vi "Process Image.vi"(8 "error in (no error)":errorcluster, 10 "Image Analysis IN":T1, 11 "Cluster in":T3={"Draw Xhair IN "={"Draw"=TRUE, "Target"={"x"=20.0, "y"=20.0}, "Size"={"x"=20.0, "y"=20.0}, "Angle"=1250067.0, "Color"=1250067, "Thickness"=20, "CrosshairLabel"=""}, "Autoscale"=FALSE, "Scale"={"scale factor"=0.0, "Scale"=FALSE}, "Lowpass IN"={"LowPass"=FALSE, "Size & Tolerance"={"X Size"=0, "Y Size"=0, "% Tolerance"=0}}, "Image"=refnum, "GUI_centroid overlay"={"CentroidX array"=[], "CentroidY array"=[], "CentroidX"=0.0, "CentroidY"=0.0, "# images to average"=1250067, "Overlay Size"={"xhair size"=0.0, "xhair size 2"=0.0}, "Color"=1250067, "Draw"=FALSE, "Thickness"=0}, "GUI Xhair"={"Draw"=TRUE, "Target"={"x"=20.0, "y"=20.0}, "Size"={"x"=20.0, "y"=20.0}, "Angle"=1250067.0, "Color"=1250067, "Thickness"=20, "CrosshairLabel"=""}} {"Draw Xhair IN"."Thickness" max=0; "Draw Xhair IN"."Target"."y" min=0.0 max=0.0; "Draw Xhair IN"."Target"."x" min=0.0 max=0.0; "Draw Xhair IN"."Angle" format="%#_13g"; "Draw Xhair IN"."Size"."y" min=0.0 max=0.0; "Draw Xhair IN"."Size"."x" min=0.0 max=0.0; "GUI Xhair"."Thickness" max=0; "GUI Xhair"."Target"."y" min=0.0 max=0.0; "GUI Xhair"."Target"."x" min=0.0 max=0.0; "GUI Xhair"."Angle" format="%#_13g"; "GUI Xhair"."Size"."y" min=0.0 max=0.0; "GUI Xhair"."Size"."x" min=0.0 max=0.0}) -> (0 "error out":errorcluster, 2 "Image Analysis OUT":T1, 3 "Cluster out":T3={"Draw Xhair IN "={"Draw"=TRUE, "Target"={"x"=20.0, "y"=20.0}, "Size"={"x"=20.0, "y"=20.0}, "Angle"=1250067.0, "Color"=1250067, "Thickness"=20, "CrosshairLabel"=""}, "Autoscale"=FALSE, "Scale"={"scale factor"=0.0, "Scale"=FALSE}, "Lowpass IN"={"LowPass"=FALSE, "Size & Tolerance"={"X Size"=0, "Y Size"=0, "% Tolerance"=0}}, "Image"=refnum, "GUI_centroid overlay"={"CentroidX array"=[], "CentroidY array"=[], "CentroidX"=0.0, "CentroidY"=0.0, "# images to average"=1250067, "Overlay Size"={"xhair size"=0.0, "xhair size 2"=0.0}, "Color"=1250067, "Draw"=FALSE, "Thickness"=0}, "GUI Xhair"={"Draw"=TRUE, "Target"={"x"=20.0, "y"=20.0}, "Size"={"x"=20.0, "y"=20.0}, "Angle"=1250067.0, "Color"=1250067, "Thickness"=20, "CrosshairLabel"=""}} {"Draw Xhair IN"."Thickness" max=0; "Draw Xhair IN"."Target"."y" min=0.0 max=0.0; "Draw Xhair IN"."Target"."x" min=0.0 max=0.0; "Draw Xhair IN"."Angle" format="%#_13g"; "Draw Xhair IN"."Size"."y" min=0.0 max=0.0; "Draw Xhair IN"."Size"."x" min=0.0 max=0.0; "GUI Xhair"."Thickness" max=0; "GUI Xhair"."Target"."y" min=0.0 max=0.0; "GUI Xhair"."Target"."x" min=0.0 max=0.0; "GUI Xhair"."Angle" format="%#_13g"; "GUI Xhair"."Size"."y" min=0.0 max=0.0; "GUI Xhair"."Size"."x" min=0.0 max=0.0})   [LabVIEW 2020]
uses:
  Controls/Image Processing Controls.ctl
  General GUIs/Device GUIs/GUI_Cameras/Controls/Crosshair type def.ctl
  <vilib>/vision/Image Controls.llb/IMAQ Image.ctl
  Controls/GUI_running average centroid overlay.ctl
  Controls/Image Analysis Controls.ctl
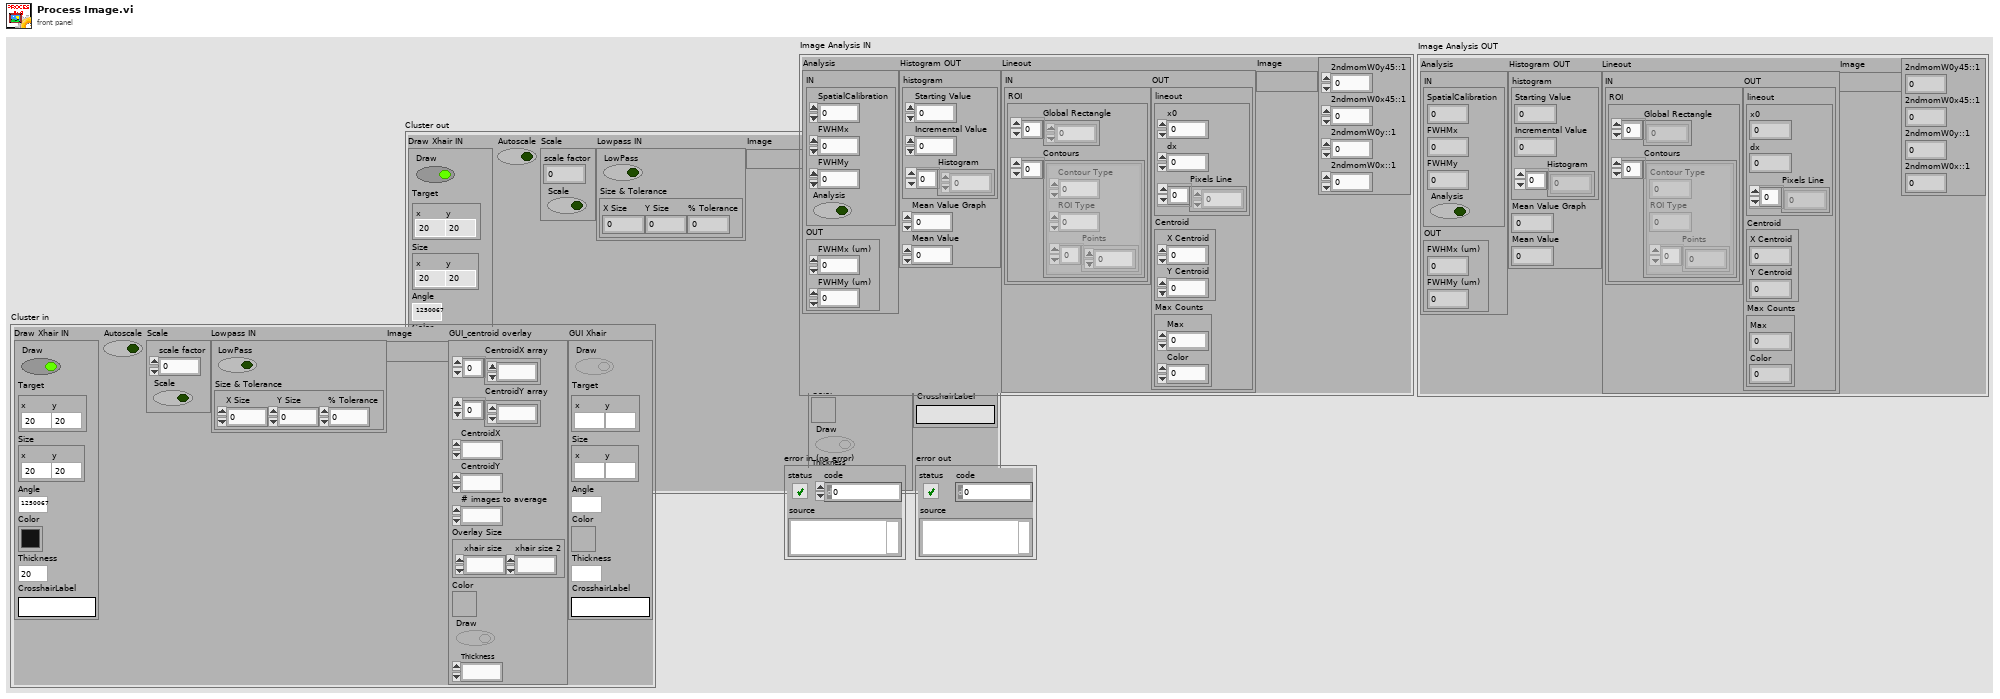
[diagram p1: front panel]
types:
  T1 = typedef "Image Analysis Controls.ctl" = cluster{"Analysis":cluster{"IN":cluster{"SpatialCalibration":dbl, "FWHMx":dbl, "FWHMy":dbl, "Analysis":bool}, "OUT":cluster{"FWHMx (um)":dbl, "FWHMy (um)":dbl}}, "Histogram OUT":cluster{"histogram":cluster{"Starting Value":sgl, "Incremental Value":sgl, "Histogram":u32[]}, "Mean Value Graph":sgl, "Mean Value":sgl}, "Lineout":cluster{"IN":cluster{"ROI":cluster{"Global Rectangle":i32[], "Contours":cluster{"Contour Type":u32, "ROI Type":u32, "Points":i32[]}[]}}, "OUT":cluster{"lineout":cluster{"x0":sgl, "dx":sgl, "Pixels Line":sgl[]}, "Centroid":cluster{"X Centroid":sgl, "Y Centroid":sgl}, "Max Counts":cluster{"Max":sgl, "Color":u32}}}, "Image":T2, "variables":cluster{"2ndmomW0y45::1":dbl, "2ndmomW0x45::1":dbl, "2ndmomW0y::1":dbl, "2ndmomW0x::1":dbl}}
  T2 = typedef "IMAQ Image.ctl" = refnum<image>
  T3 = typedef "Image Processing Controls.ctl" = cluster{"Draw Xhair IN ":T4, "Autoscale":bool, "Scale":cluster{"scale factor":dbl, "Scale":bool}, "Lowpass IN":cluster{"LowPass":bool, "Size & Tolerance":cluster{"X Size":i32, "Y Size":i32, "% Tolerance":i32}}, "Image":T2, "GUI_centroid overlay":T5, "GUI Xhair":T4}
  T4 = typedef "Crosshair type def.ctl" = cluster{"Draw":bool, "Target":cluster{"x":dbl, "y":dbl}, "Size":cluster{"x":dbl, "y":dbl}, "Angle":dbl, "Color":u32, "Thickness":u8, "CrosshairLabel":string}
  T5 = typedef "GUI_running average centroid overlay.ctl" = cluster{"CentroidX array":dbl[], "CentroidY array":dbl[], "CentroidX":dbl, "CentroidY":dbl, "# images to average":i32, "Overlay Size":cluster{"xhair size":dbl, "xhair size 2":dbl}, "Color":u32, "Draw":bool, "Thickness":u8}
  T6 = cluster{"LowPass":bool, "Size & Tolerance":cluster{"X Size":i32, "Y Size":i32, "% Tolerance":i32}}
  T7 = cluster{"SpatialCalibration":dbl, "FWHMx":dbl, "FWHMy":dbl, "Analysis":bool}
  T8 = cluster{"ROI":cluster{"Global Rectangle":i32[], "Contours":cluster{"Contour Type":u32, "ROI Type":u32, "Points":i32[]}[]}}
  T9 = cluster{"histogram":cluster{"Starting Value":sgl, "Incremental Value":sgl, "Histogram":u32[]}, "Mean Value Graph":sgl, "Mean Value":sgl}
  T10 = cluster{"lineout":cluster{"x0":sgl, "dx":sgl, "Pixels Line":sgl[]}, "Centroid":cluster{"X Centroid":sgl, "Y Centroid":sgl}, "Max Counts":cluster{"Max Value":sgl, "Color":u32}}
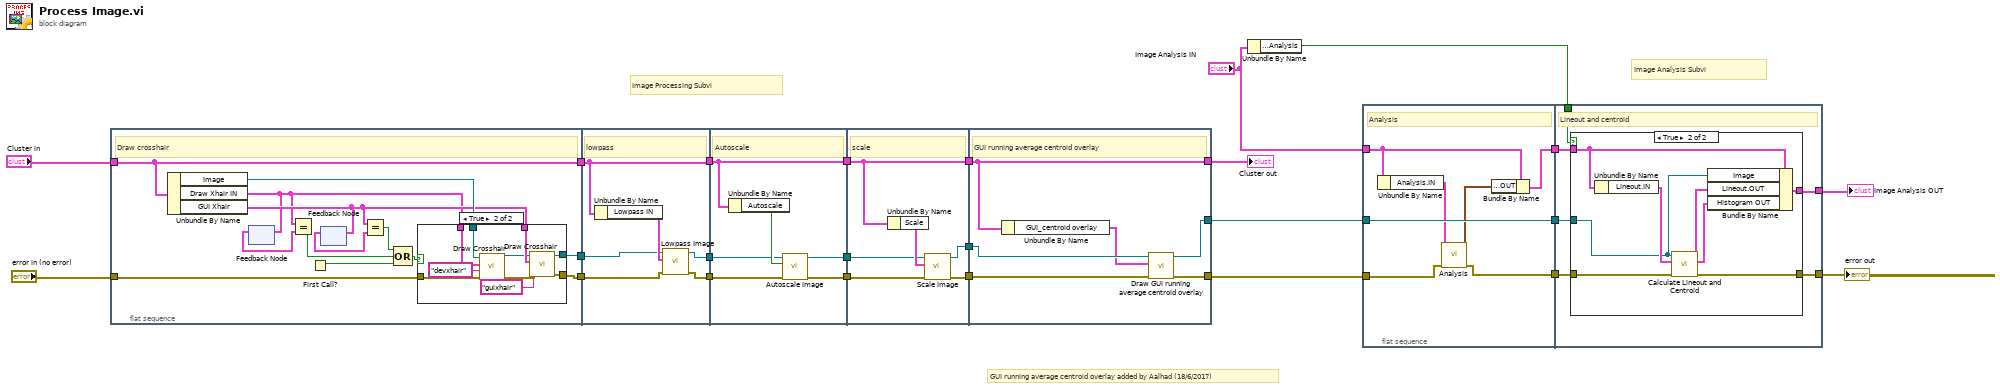
[diagram p0: block diagram]
diagram:
  # "GUI running average centroid overlay added by Aalhad (18/6/2017)"
  # "Image Analysis Subvi"
  # "Image Processing Subvi"
  n1 = flat-sequence {
    tunnel: [w37] -> w18
    tunnel: [w33] -> w17
    tunnel: [w34] -> w11
    tunnel: "Cluster in" -> [w37]
    tunnel: "error in (no error)" -> [w35]
    tunnel: [w54] -> w24
    tunnel: [w51] -> w23
    tunnel: w18 -> [w54]
    tunnel: w17 -> [w50]
    tunnel: w11 -> [w53]
    tunnel: [w52] -> w10
    tunnel: w24 -> [w56]
    tunnel: [w56] -> w22
    tunnel: w23 -> [w60]
    tunnel: [w59] -> w21
    tunnel: w10 -> [w57]
    tunnel: [w58] -> w9
    tunnel: w22 -> [w63]
    tunnel: w21 -> [w66]
    tunnel: w9 -> [w62]
    tunnel: [w63] -> w7
    tunnel: [w65] -> w6
    tunnel: [w64] -> w5
    tunnel: [w73] -> w15
    tunnel: [w72] -> w14
    tunnel: [w70] -> w20
    tunnel: w7 -> [w70]
    tunnel: w6 -> [w71]
    tunnel: w5 -> [w69]
    frame #0 {
      # "Draw crosshair"
      n2 = Unbundle By Name(w37) -> ("Image"=w36:T2, "Draw Xhair IN"=w27:T4, "GUI Xhair"=w29:T4)
      n3 = feedback #1() -> (w28:T4)  [unwired: 1 in]
      n4 = feedback-in #1(w27) -> ()
      n5 = Equal?(x=w27, y=w28) -> (x = y?=w25:bool)
      n6 = First Call?() -> (First Call?: T/F=w31:bool)
      n7 = feedback #2() -> (w32:T4)  [unwired: 1 in]
      n8 = feedback-in #2(w29) -> ()
      n9 = Equal?(x=w29, y=w32) -> (x = y?=w26:bool)
      n10 = Compound Arithmetic op=OR(w26, w25, w31) -> (w30:bool)
      n11 = case shown="True" w30 {
        tunnel: w27 -> [_ w49]
        tunnel: w36 -> [w38 w48]
        tunnel: w35 -> [w39 w47]
        tunnel: w29 -> [_ w46]
        tunnel: [w38 w43] -> w34
        tunnel: [w39 w42] -> w33
        frame False {
        }
        frame True {
          n12 = call "Draw Crosshair.vi"("error in"=w47, "xhair name"="devxhair", "Crosshair"=w49, "Image in"=w48) -> ("error out"=w44:errorcluster, "image out"=w45:T2)  [unwired: 6 in]
          n13 = call "Draw Crosshair.vi"("error in"=w44, "xhair name"="guixhair", "Crosshair"=w46, "Image in"=w45) -> ("error out"=w42:errorcluster, "image out"=w43:T2)  [unwired: 6 in]
        }
      }
    }
    frame #1 {
      # "lowpass"
      n14 = Unbundle By Name(w54) -> ("Lowpass IN"=w55:T6)
      n15 = call "Lowpass Image.vi"("error in"=w50, "Lowpass IN"=w55, "Refnum in"=w53) -> ("error out"=w51:errorcluster, "Refnum out"=w52:T2)  [unwired: 7 in]
    }
    frame #2 {
      # "Autoscale"
      n16 = Unbundle By Name(w56) -> ("Autoscale"=w61:bool)
      n17 = call "Autoscale Image.vi"("error in (no error)"=w60, "Autoscale"=w61, "Refnum in"=w57) -> ("error out"=w59:errorcluster, "Refnum out"=w58:T2)  [unwired: 7 in]
    }
    frame #3 {
      # "scale"
      n18 = Unbundle By Name(w63) -> ("Scale"=w67:cluster{"scale factor":dbl, "Scale":bool})
      n19 = call "Scale Image.vi"("error in (no error)"=w66, "Scale"=w67, "Refnum in"=w62) -> ("error out"=w65:errorcluster, "Refnum out"=w64:T2)  [unwired: 7 in]
    }
    frame #4 {
      # "GUI running average centroid overlay"
      n20 = Unbundle By Name(w70) -> ("GUI_centroid overlay"=w68:T5)
      n21 = call "Draw GUI running average centroid overlay.vi"("error in"=w71, "GUI_centroid overlay"=w68, "Image in"=w69) -> ("error out"=w72:errorcluster, "image out"=w73:T2)  [unwired: 7 in]
    }
  }
  n22 = Unbundle By Name("Image Analysis IN") -> ("Analysis.IN.Analysis"=w1:bool)
  n23 = flat-sequence {
    tunnel: w14 -> [w78]
    tunnel: w15 -> [w80]
    tunnel: "Image Analysis IN" -> [w76]
    tunnel: [w75] -> w4
    tunnel: [w80] -> w3
    tunnel: [w77] -> w2
    tunnel: w4 -> [w84]
    tunnel: w3 -> [w86]
    tunnel: w2 -> [w85]
    tunnel: [w83] -> w12
    tunnel: [w82] -> w13
    tunnel: w1 -> [w81]
    frame #0 {
      # "Analysis"
      n24 = Unbundle By Name(w76) -> ("Analysis.IN"=w79:T7)
      n25 = call "Analysis.vi"("error in"=w78, "IN"=w79) -> ("error out"=w77:errorcluster, "OUT"=w74:cluster{"FWHMx (um)":dbl, "FWHMy (um)":dbl})  [unwired: 8 in]
      n26 = Bundle By Name(cluster=w76, "Analysis.OUT"=w74) -> (w75:T1)
    }
    frame #1 {
      # "Lineout and centroid"
      n27 = case shown="True" w81 {
        tunnel: w86 -> [_ w94]
        tunnel: w85 -> [w88 w93]
        tunnel: w84 -> [w87 w92]
        tunnel: [w87 w90] -> w83
        tunnel: [w88 w89] -> w82
        frame False {
        }
        frame True {
          n28 = Unbundle By Name(w92) -> ("Lineout.IN"=w96:T8)
          n29 = call "Calculate Lineout and Centroid.vi"("error in (no error)"=w93, "Lineout IN"=w96, "Image"=w94) -> ("error out"=w89:errorcluster, "Histogram OUT"=w91:T9, "Lineout Out"=w95:T10)  [unwired: 6 in]
          n30 = Bundle By Name(cluster=w92, "Image"=w94, "Lineout.OUT"=w95, "Histogram OUT"=w91) -> (w90:T1)
        }
      }
    }
  }
  "Cluster out" <- w20
  "error out" <- w13
  "Image Analysis OUT" <- w12
